vi "TestPage1.vi"() -> ()   [LabVIEW 2013]
panel:
  out "x+y":dbl
  in  "OK Button":bool
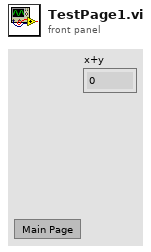
[diagram p1: front panel]
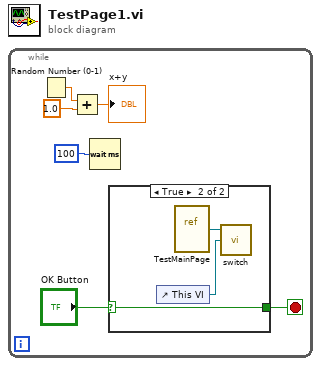
[diagram p0: block diagram]
diagram:
  n1 = while {
    stop <- w6 stop-if-true
    n2 = Random Number (0-1)() -> (number: 0 to 1=w1:dbl)
    n3 = Add(x=w1, y=1.0) -> (x+y=→"x+y":dbl)
    n4 = Wait (ms)(milliseconds to wait=u32 100) -> ()  [unwired: 1 out]
    n5 = case shown="True" "OK Button" {
      selector: "OK Button" -> [_ w7]
      tunnel: [_ w7] -> w6
      frame False {
      }
      frame True {
        n6 = control-ref of="This VI"() -> (w8:refnum<vi>)
        n7 = vi-ref "TestMainPage.vi"() -> (w9:refnum<vi>)
        n8 = call "switch.vi"("vi close"=w8, "vi open"=w9) -> ()  [unwired: 1 in, 1 out]
      }
    }
  }
